vi "GKC-1_Verileri.vi"() -> ()   [LabVIEW 2014]
uses:
  CustomControls/TSE_Status.ctl
  CustomControls/Program_States.ctl
panel:
  in  "GKÇ-1 Test Status":T1={"Return Code"=0, "Message"="", "error in (no error)"={"status"=FALSE, "code"=0, "source"=""}, "Program State"=enum."Ön Yükleme Tamam", "Test A. Suresi"=0}
  in  "GKÇ-1 Tip":enum16{"", "PQ+", "PQ++", "ION"}(ring)
  in  "GKÇ-1 IP Adresi":string
  in  "GKÇ-1 Seri No":string
  in  "FD2 C Fazı Harmonik Ölçüm Değerleri":dbl[](array[numeric])
  in  "FD2 B Fazı Harmonik Ölçüm Değerleri":dbl[](array[numeric])
  in  "FD2 A Fazı Harmonik Ölçüm Değerleri":dbl[](array[numeric])
  in  "FD1 C Fazı Harmonik Ölçüm Değerleri":dbl[](array[numeric])
  in  "FD1 B Fazı Harmonik Ölçüm Değerleri":dbl[](array[numeric])
  in  "FD1 A Fazı Harmonik Ölçüm Değerleri":dbl[](array[numeric])
  in  "Harmonik Limit Değerler":dbl[](array[numeric])
  in  "Uygulanan Değerler":dbl[](array[numeric])
  in  "Uygulanan Değer":dbl
  in  "FD2 C":dbl
  in  "FD2 B":dbl
  in  "FD2 A":dbl
  in  "FD1 C":dbl
  in  "FD1 B":dbl
  in  "FD1 A":dbl
  in  "Limit Deger":dbl
  in  "Ölçüm No":u16
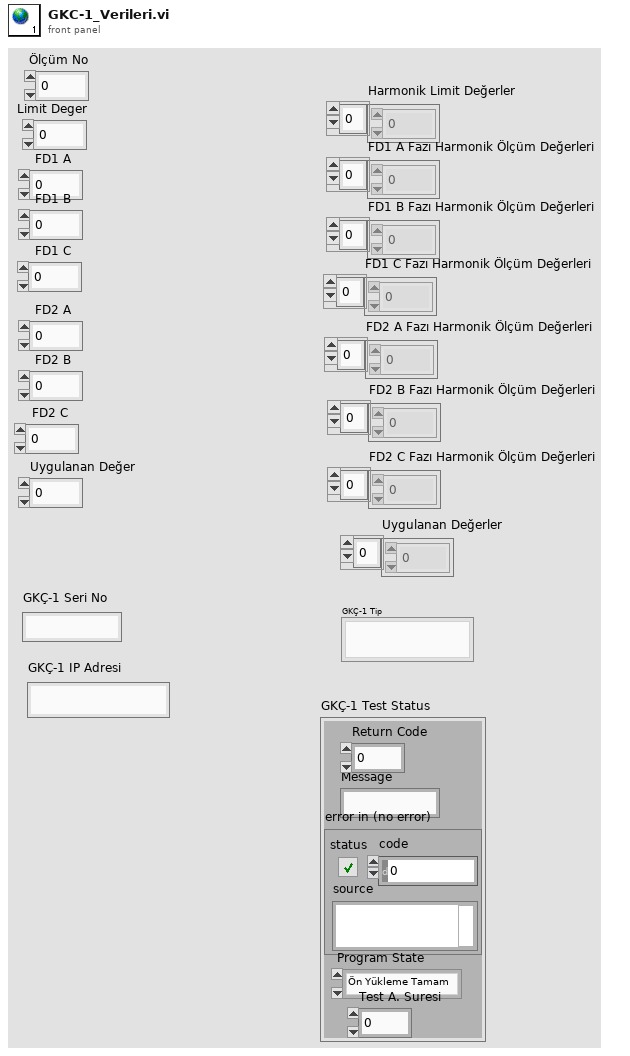
[diagram p1: front panel]
types:
  T1 = typedef "TSE_Status.ctl" = cluster{"Return Code":i32, "Message":string, "error in (no error)":errorcluster, "Program State":T2, "Test A. Suresi":u32}
  T2 = typedef "Program_States.ctl" = enum16{"Ön Yükleme", "TSE Baslat", "Kalibratöre Baglan", "Kalibratörü Baslat", "Ön Yükleme Tamam", "Frekans Testi", "Gerilim Testi", "Akim Testi", "Aktif Guc Testi", "Reaktif Guc Testi", "AC Akim Harmonik Testi", "AC Gerilim Harmonik Testi", "Flicker Testi", "Rapor Cikarma", "Yeniden Başlat", "Bekleme", "Durdur"}
diagram:
